vi "svx_Colormap Order Lines Line Property Color write.vi"(4 "error in (no error)":errorcluster, 5 "Value":u32, 6 "Container State":T2, 7 "Display State In":T1={"RefQueue"=refnum, "Properties/Undo"=refnum, "Bound"={"Width"=0, "Height"=0}, "Plot Area:Colors"={"FG Color"=11776947, "BG Color"=0}, "scale legend visible?"=FALSE, "graph palette visible?"=FALSE, "cursor palette visible?"=FALSE, "Ignore Array"=TRUE, "Smooth Update"=FALSE, "Z Scale"={"Z Scale.Scale Fit"=2, "Z Scale.Name Label.Text"="Amplitude", "Z Scale.Interpolate Color"=TRUE, "Visible"=TRUE, "Label Visible"=TRUE, "format string"="%#.2g", "Z Scale.Range"={"Minimum"=0.0, "Maximum"=500.0}}, "X Scale"={"X Scale.Scale Fit"=2, "X Scale.Offset and Multiplier"={"Offset"=0.0, "Multiplier"=1.0}, "X Scale.Name Label.Text"="Time", "X Scale.Range"={"Minimum"=0.0, "Maximum"=10.0}, "Visible"=TRUE, "Label Visible"=TRUE, "format string"="%#.2g"}, "Y Scale"={"Y Scale.Scale Fit"=2, "Y Scale.Offset and Multiplier"={"Offset"=0.0, "Multiplier"=1.0}, "Y Scale.Name Label.Text"="Frequency", "Y Scale.Range"={"Minimum"=0.0, "Maximum"=500.0}, "Visible"=TRUE, "Label Visible"=TRUE, "format string"="%#.2g"}, "Annotation List"=[], "Cursor List"=[], "Display Frequency Lines"=TRUE, "Display Order Lines"=TRUE, "Display Order text"=TRUE, "Display Frequency text"=TRUE, "Order Lineproperty"={"Line"={"Width"=1, "Style"=enum."Dash"}, "color"=0}, "Order Textproperty"={"Test size"=11, "color"=16777222, "background"=16777216}, "Orders"=[], "Frequency"=[], "Frequency Lineproperty"={"Line"={"Width"=1, "Style"=enum."Dash"}, "color"=0}, "Frequency Textproperty"={"Test size"=11, "color"=16777222, "background"=16777216}, "Display Order from Cursor"=FALSE, "Display Freq from Cursor"=FALSE, "Active Cursor"=0, "Selected Cursors"=[], "Cursor Move"=refnum, "Scale Range Change"=refnum}) -> (0 "error out":errorcluster, 3 "Display State Out":T1={"RefQueue"=refnum, "Properties/Undo"=refnum, "Bound"={"Width"=0, "Height"=0}, "Plot Area:Colors"={"FG Color"=11776947, "BG Color"=0}, "scale legend visible?"=FALSE, "graph palette visible?"=FALSE, "cursor palette visible?"=FALSE, "Ignore Array"=TRUE, "Smooth Update"=FALSE, "Z Scale"={"Z Scale.Scale Fit"=2, "Z Scale.Name Label.Text"="Amplitude", "Z Scale.Interpolate Color"=TRUE, "Visible"=TRUE, "Label Visible"=TRUE, "format string"="%#.2g", "Z Scale.Range"={"Minimum"=0.0, "Maximum"=500.0}}, "X Scale"={"X Scale.Scale Fit"=2, "X Scale.Offset and Multiplier"={"Offset"=0.0, "Multiplier"=1.0}, "X Scale.Name Label.Text"="Time", "X Scale.Range"={"Minimum"=0.0, "Maximum"=10.0}, "Visible"=TRUE, "Label Visible"=TRUE, "format string"="%#.2g"}, "Y Scale"={"Y Scale.Scale Fit"=2, "Y Scale.Offset and Multiplier"={"Offset"=0.0, "Multiplier"=1.0}, "Y Scale.Name Label.Text"="Frequency", "Y Scale.Range"={"Minimum"=0.0, "Maximum"=500.0}, "Visible"=TRUE, "Label Visible"=TRUE, "format string"="%#.2g"}, "Annotation List"=[], "Cursor List"=[], "Display Frequency Lines"=TRUE, "Display Order Lines"=TRUE, "Display Order text"=TRUE, "Display Frequency text"=TRUE, "Order Lineproperty"={"Line"={"Width"=1, "Style"=enum."Dash"}, "color"=0}, "Order Textproperty"={"Test size"=11, "color"=16777222, "background"=16777216}, "Orders"=[], "Frequency"=[], "Frequency Lineproperty"={"Line"={"Width"=1, "Style"=enum."Dash"}, "color"=0}, "Frequency Textproperty"={"Test size"=11, "color"=16777222, "background"=16777216}, "Display Order from Cursor"=FALSE, "Display Freq from Cursor"=FALSE, "Active Cursor"=0, "Selected Cursors"=[], "Cursor Move"=refnum, "Scale Range Change"=refnum})   [LabVIEW 2017, in "SVX Colormap.xctl"]
uses:
  <vilib>/addons/_XControls/Colormap/SVX Colormap.xctl
  <vilib>/_xctls/Container State.ctl
  <vilib>/addons/_XControls/Colormap/subVIs/svx_Colormap State.ctl
  <vilib>/addons/_XControls/Colormap/TypeDef/svx_Colormap_InnerState.ctl
  <vilib>/addons/_XControls/Colormap/TypeDef/svx_Colormap_Event.ctl
  <vilib>/_xctls/XControlSupport.lvlib
panel:
  # "Replace the Value Control below with a Control of desired type.\nDo not remove this Control or the others from the connector pane.\nDo not change the connector pane pattern.\nThe Value control should always be the third terminal from top on the input side in the connector pane."
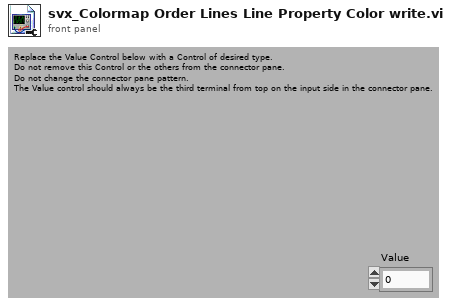
[diagram p1: front panel]
types:
  T1 = typedef "SVX Colormap.xctl/svx_Colormap State.ctl" = cluster{"RefQueue":refnum<queue>, "Properties/Undo":refnum<queue>, "Bound":cluster{"Width":u32, "Height":u32}, "Plot Area:Colors":cluster{"FG Color":u32, "BG Color":u32}, "scale legend visible?":bool, "graph palette visible?":bool, "cursor palette visible?":bool, "Ignore Array":bool, "Smooth Update":bool, "Z Scale":cluster{"Z Scale.Scale Fit":u8, "Z Scale.Name Label.Text":string, "Z Scale.Interpolate Color":bool, "Visible":bool, "Label Visible":bool, "format string":string, "Z Scale.Range":cluster{"Minimum":dbl, "Maximum":dbl}}, "X Scale":cluster{"X Scale.Scale Fit":u8, "X Scale.Offset and Multiplier":cluster{"Offset":dbl, "Multiplier":dbl}, "X Scale.Name Label.Text":string, "X Scale.Range":cluster{"Minimum":dbl, "Maximum":dbl}, "Visible":bool, "Label Visible":bool, "format string":string}, "Y Scale":cluster{"Y Scale.Scale Fit":u8, "Y Scale.Offset and Multiplier":cluster{"Offset":dbl, "Multiplier":dbl}, "Y Scale.Name Label.Text":string, "Y Scale.Range":cluster{"Minimum":dbl, "Maximum":dbl}, "Visible":bool, "Label Visible":bool, "format string":string}, "Annotation List":cluster{"Name":string, "Color":u32, "Style":u8, "Point Style":u8, "Name Visible":bool, "Allow Drag":bool, "Annotation Mode":u32, "Plot":i32, "Index":i32, "Position":cluster{"X":dbl, "Y":dbl}, "X Scale":u32, "Y Scale":u32, "Show Arrow":bool, "Lock Name":bool, "Plot Area":i32, "Label Offset":cluster{"X":dbl, "Y":dbl}}[], "Cursor List":cluster{"Name":string, "Color":u32, "Style":u8, "Point Style":u8, "Name Visible":bool, "Allow Drag":bool, "Cursor Mode":u32, "Plot":i32, "Index":i32, "Position":cluster{"X":dbl, "Y":dbl}, "X Scale":u32, "Y Scale":u32, "Watch Plots":i32[], "Watch All Plots":bool, "Plot Area":i32, "Label Offset":cluster{"X":dbl, "Y":dbl}}[], "Display Frequency Lines":bool, "Display Order Lines":bool, "Display Order text":bool, "Display Frequency text":bool, "Order Lineproperty":cluster{"Line":cluster{"Width":u16, "Style":enum32{"Solid", "Dash", "Dot", "DashDot", "DashDotDot"}}, "color":u32}, "Order Textproperty":cluster{"Test size":i16, "color":u32, "background":u32}, "Orders":dbl[], "Frequency":dbl[], "Frequency Lineproperty":cluster{"Line":cluster{"Width":u16, "Style":enum32{"Solid", "Dash", "Dot", "DashDot", "DashDotDot"}}, "color":u32}, "Frequency Textproperty":cluster{"Test size":i16, "color":u32, "background":u32}, "Display Order from Cursor":bool, "Display Freq from Cursor":bool, "Active Cursor":u32, "Selected Cursors":u32[], "Cursor Move":refnum<user-event>, "Scale Range Change":refnum<user-event>}
  T2 = typedef "XControlSupport.lvlib/Container State.ctl" = cluster{"Indicator?":bool, "Run Mode?":bool, " Refnum":refnum<vi>}
  T3 = typedef "SVX Colormap.xctl/svx_Colormap_Event.ctl" = enum16{"None", "[Axis] X Range", "[Axis] Y Range", "[Axis] Z Range", "[Axis] Range", "[Axis] X FString", "[Axis] Y FString", "[Axis] Z FString", "[Axis] X Name", "[Axis] X ScaleVis", "[Axis] X NameVis", "[Axis] Y Name", "[Axis] Y ScaleVis", "[Axis] Y NameVis", "[Axis] Z Name", "[Axis] Z ScaleVis", "[Axis] Z NameVis", "[Image] Line", "[Axis] Z Interp", "[Data] Update", "[Layout] Resize", "[ColorTable] Ignore Array", "[Legend] ScaleVis", "[Legend] GPVis", "[Legend] CPVis", "[Smooth] Update", "[Cursor] Update", "[Plot Area] Colors", "[Size] Minimum", "[Annotation] Update", "[Properties Dialog]", "[Axis] Autoscale X", "[Axis] Autoscale Y", "[Axis] Autoscale Z"}
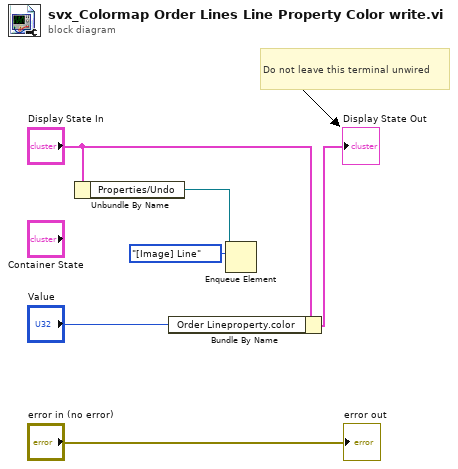
[diagram p0: block diagram]
diagram:
  # "Do not leave this terminal unwired"
  n1 = Unbundle By Name("Display State In") -> ("Properties/Undo"=w2:refnum<queue>)
  n2 = Bundle By Name(cluster="Display State In", "Order Lineproperty.color"="Value") -> (→"Display State Out":T1)
  n3 = Enqueue Element(queue=w2, element=svx_Colormap_Event."[Image] Line") -> ()  [unwired: 2 in, 3 out]
  "error out" <- "error in (no error)"
